vi "ICM Parsing Logic.vi"(8 "error in (no error)":errorcluster, 10 "Data String":string, 11 "Format String":string) -> (0 "error out":errorcluster, 3 "Data Values":dbl[](array[numeric]))   [LabVIEW 2018]
doc: "ICM Parsing Logic.vi\n\nThis VI includes the parsing functionality built into LabVIEW and custom parsing written for ICM. It is used by the ICM General Parser and the ICM Multi-Sentence Parser.\n\nInstrument Communication Module Version 1.0\nDecember, 2020 Original Code Consulting David Thomson\n www.originalcode.com"
uses:
  Parsing VIs/ICM whitespace.ctl
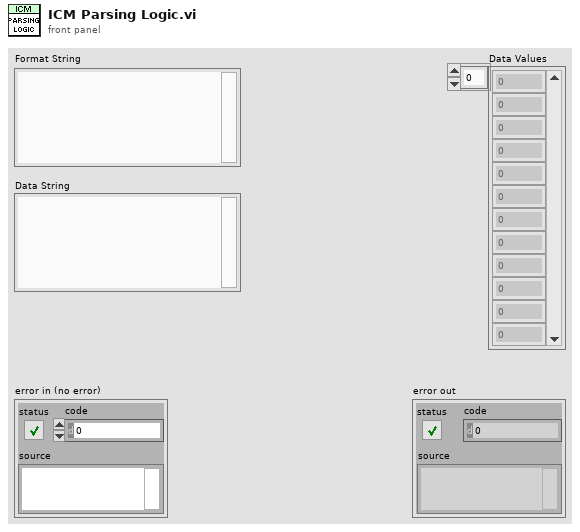
[diagram p1: front panel]
types:
  T1 = typedef "ICM whitespace.ctl" = u16
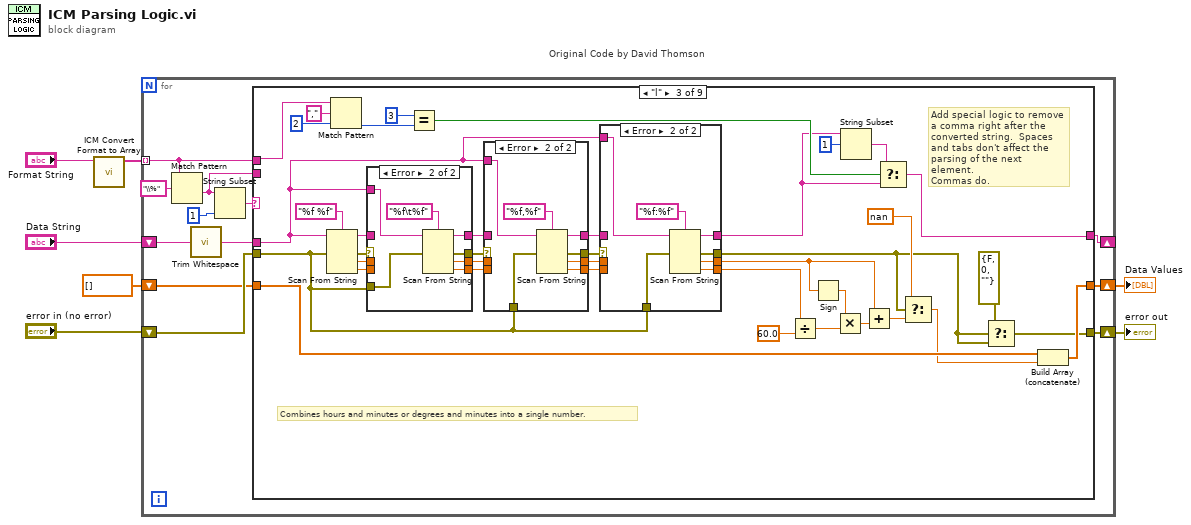
[diagram p0: block diagram]
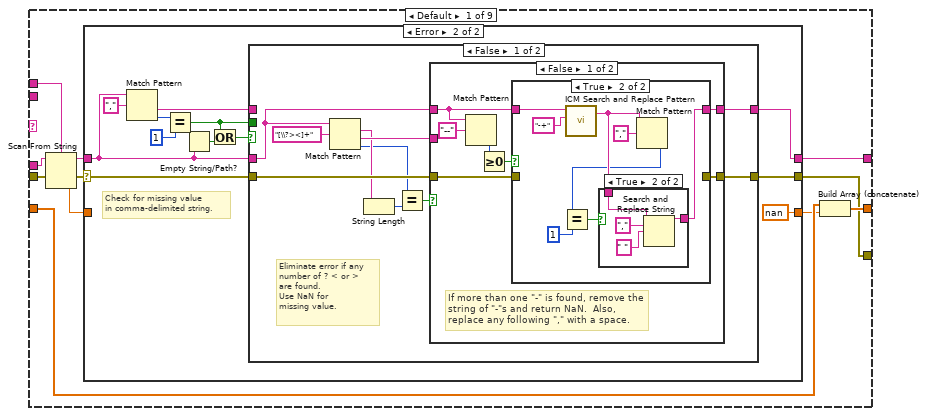
[diagram p2: hidden frame]
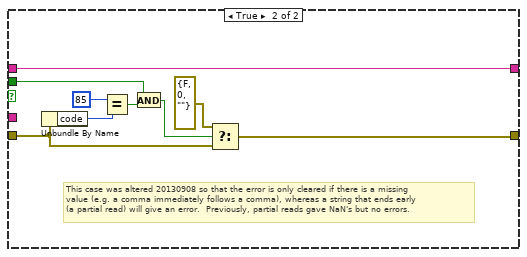
[diagram p7: hidden frame]
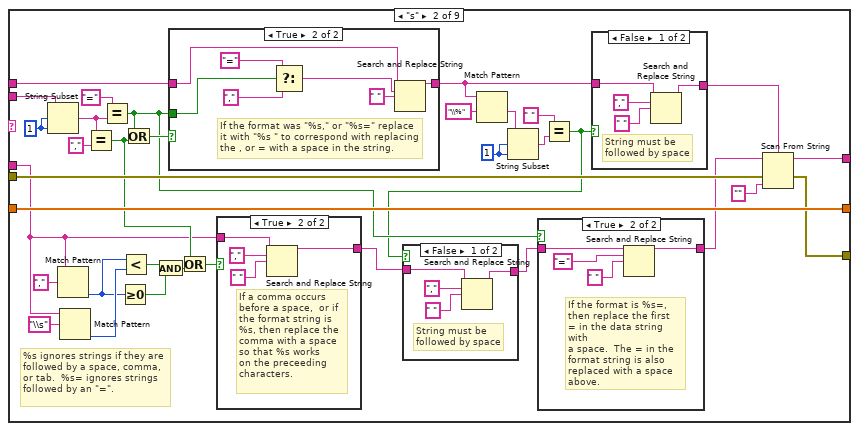
[diagram p8: hidden frame]
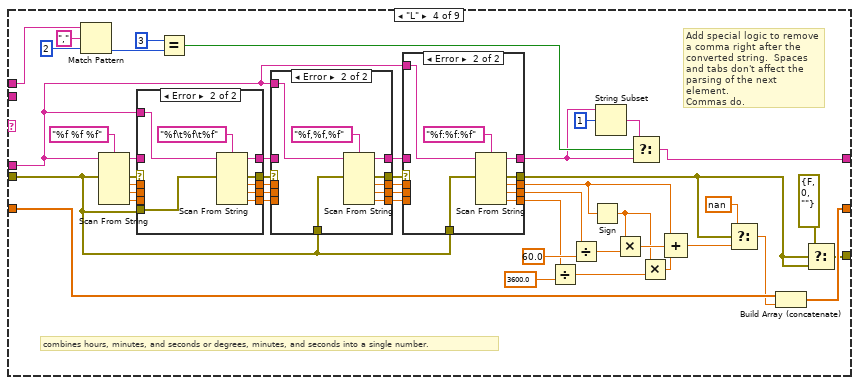
[diagram p17: hidden frame]
diagram:
  n1 = call "ICM Convert Format to Array.vi"("Format String"="Format String") -> ("Format Array"=w7:string[])  [unwired: 10 in]
  n2 = for "Original Code by David Thomson" {
    shift-right: [w13] -> _
    shift-left: "Data String" -> [w9]
    shift-right: [w14] -> w2
    shift-left: "error in (no error)" -> [w19]
    tunnel: w7 -> [w11] mode=indexing
    shift-right: [w16] -> w5
    shift-left: dbl[] [] -> [w17]
    n3 = Match Pattern(string=w11, regular expression="\\%") -> (after substring=w10:string)  [unwired: 4 out]
    n4 = call <vilib>:"Trim Whitespace.vi"("string"=w9) -> ("trimmed string"=w8:string)  [unwired: 1 in]
    n5 = String Subset(string=w10, length (rest)=1 ("length (rest)")) -> (substring=w15:string)  [unwired: 1 out]
    n6 = case shown="\"l\"" w15 {
      selector: w15 -> [_ _ _ _ _ w347 _ _ _]
      tunnel: w19 -> [w30 w118 w155 w230 w326 w355 w441 w459 w557]
      tunnel: w11 -> [w29 w108 w170 w240 _ _ _ _ _]
      tunnel: [w28 w119 w182 w262 w324 w339 w443 w460 w555] -> w16
      tunnel: w17 -> [w23 w119 w183 w263 w325 _ w443 w461 w572]
      tunnel: [w26 w117 w160 w234 w322 w348 w441 w458 w558] -> w14
      tunnel: [w21 w121 w165 w236 w323 w349 w442 w463 w551] -> w13
      tunnel: w10 -> [_ w110 _ _ w310 _ w437 w457 w565]
      tunnel: w8 -> [w20 w88 w150 w222 w307 w336 w429 w448 w550]
      frame Default {
        n7 = Scan From String(format string=w29, input string=w20, error in=w30) -> (remaining string=w25:string, error out=w27:errorcluster, output 1=w24:dbl)  [unwired: 1 in, 2 out]
        n8 = case shown="Error" w27 {
          selector: w27 -> [w33 w41]
          tunnel: [w33 w35] -> w26
          tunnel: [w32 w36] -> w21
          tunnel: w25 -> [w32 w37]
          tunnel: w24 -> [w31 _]
          tunnel: [w31 nan ("y")] -> w22
          frame No Error {
            # "this case uses LabVIEW's built in parsing codes"
          }
          frame Error {
            # "Check for missing value\nin comma-delimited string."
            n9 = Match Pattern(string=w37, regular expression=",") -> (after substring=w42:string, offset past match=w44:i32)  [unwired: 3 out]
            n10 = Equal?(x=w44, y=1) -> (x = y?=w34:bool)
            n11 = Empty String/Path?(string/path=w37) -> (empty?=w38:bool)
            n12 = Or(x=w34, y=w38) -> (x .or. y?=w39:bool)
            n13 = case shown="False" w39 {
              tunnel: [w51 w87] -> w36
              tunnel: w42 -> [_ w87]
              tunnel: w37 -> [w53 _]
              tunnel: [w50 w86] -> w35
              tunnel: w41 -> [w52 w85]
              tunnel: w34 -> [_ w80]
              frame False {
                # "Eliminate error if any\nnumber of ? < or >\nare found.\nUse NaN for\nmissing value."
                n14 = Match Pattern(string=w53, regular expression="[\\?><]+") -> (match substring=w48:string, after substring=w49:string, offset past match=w46:i32)  [unwired: 2 out]
                n15 = String Length(string=w48) -> (length=w47:i32)
                n16 = Equal?(x=w46, y=w47) -> (x = y?=w54:bool)
                n17 = case shown="False" w54 {
                  tunnel: [w57 w78] -> w51
                  tunnel: w53 -> [w56 _]
                  tunnel: [w58 _] -> w50
                  tunnel: w52 -> [w59 _]
                  tunnel: w49 -> [_ w78]
                  frame False {
                    # "If more than one \"-\" is found, remove the\nstring of \"-\"s and return NaN.  Also,\nreplace any following \",\" with a space."
                    n18 = Match Pattern(string=w56, regular expression="--") -> (offset past match=w61:i32)  [unwired: 4 out]
                    n19 = Greater Or Equal To 0?(x=w61) -> (x >= 0?=w60:bool)
                    n20 = case shown="True" w60 {
                      tunnel: [w64 _] -> w58
                      tunnel: w59 -> [w64 _]
                      tunnel: [w63 w70] -> w57
                      tunnel: w56 -> [w63 w72]
                      frame False {
                      }
                      frame True {
                        n21 = call "ICM Search and Replace Pattern.vi"("string"=w72, "regular expression (\"\")"="-+" ("regular expression (\"\")")) -> ("result string"=w68:string)  [unwired: 1 in, 3 out]
                        n22 = Match Pattern(string=w68, regular expression=",") -> (offset past match=w66:i32)  [unwired: 4 out]
                        n23 = Equal?(x=w66, y=1) -> (x = y?=w65:bool)
                        n24 = case shown="True" w65 {
                          tunnel: w68 -> [w73 w75]
                          tunnel: [w73 w74] -> w70
                          frame False {
                          }
                          frame True {
                            n25 = Search and Replace String(input string=w75, search string=",", replace string=" " ("replace string (\"\")")) -> (result string=w74:string)  [unwired: 1 in, 7 out]
                          }
                        }
                      }
                    }
                  }
                  frame True {
                  }
                }
              }
              frame True {
                # "This case was altered 20130908 so that the error is only cleared if there is a missing\nvalue (e.g. a comma immediately follows a comma), whereas a string that ends early\n(a partial read) will give an error.  Previously, partial reads gave NaN's but no errors."
                n26 = Unbundle By Name(w85) -> ("code"=w84:i32)
                n27 = Equal?(x=85, y=w84) -> (x = y?=w81:bool)
                n28 = And(x=w80, y=w81) -> (x .and. y?=w79:bool)
                n29 = Select(t=errorcluster {"status"=FALSE, "code"=0, "source"=""}, s=w79, f=w85) -> (s? t:f=w86:errorcluster)
              }
            }
          }
        }
        n30 = Build Array (concatenate)(w23, w22) -> (w28:dbl[])
      }
      frame "s" {
        w94 = 1 ("length (rest)")
        w107 = 1 ("length (rest)")
        # "%s ignores strings if they are\nfollowed by a space, comma,\nor tab.  %s= ignores strings followed by an \"=\"."
        n31 = String Subset(string=w110, offset (0)=w107, length (rest)=w107) -> (substring=w105:string)
        n32 = Match Pattern(string=w88, regular expression=",") -> (offset past match=w112:i32)  [unwired: 4 out]
        n33 = Match Pattern(string=w88, regular expression="\\s") -> (offset past match=w114:i32)  [unwired: 4 out]
        n34 = Equal?(x=w105, y=",") -> (x = y?=w100:bool)
        n35 = Equal?(x="=" ("y"), y=w105) -> (x = y?=w102:bool)
        n36 = Greater Or Equal To 0?(x=w112) -> (x >= 0?=w111:bool)
        n37 = Less?(x=w112, y=w114) -> (x < y?=w113:bool)
        n38 = Or(x=w102, y=w100) -> (x .or. y?=w106:bool)
        n39 = And(x=w113, y=w111) -> (x .and. y?=w101:bool)
        n40 = case shown="True" w106 {
          tunnel: [w137 w142] -> w93
          tunnel: w108 -> [w137 w143]
          tunnel: w102 -> [_ w138]
          frame False {
          }
          frame True {
            # "If the format was \"%s,\" or \"%s=\" replace\nit with \"%s \" to correspond with replacing\nthe , or = with a space in the string."
            n41 = Select(t="=" ("y"), s=w138, f="," ("search string")) -> (s? t:f=w139:string)
            n42 = Search and Replace String(input string=w143, search string=w139, replace string=" " ("replace string (\"\")")) -> (result string=w142:string)  [unwired: 1 in, 7 out]
          }
        }
        n43 = Or(x=w100, y=w101) -> (x .or. y?=w99:bool)
        n44 = case shown="True" w99 {
          tunnel: [w145 w147] -> w91
          tunnel: w88 -> [w145 w146]
          frame False {
          }
          frame True {
            # "If a comma occurs\nbefore a space,  or if\nthe format string is %s, then replace the comma with a space so that %s works\non the preceeding characters."
            n45 = Search and Replace String(input string=w146, search string=",", replace string=" " ("replace string (\"\")")) -> (result string=w147:string)  [unwired: 1 in, 7 out]
          }
        }
        n46 = Match Pattern(string=w93, regular expression="\\%") -> (after substring=w95:string)  [unwired: 4 out]
        n47 = String Subset(string=w95, offset (0)=w94, length (rest)=w94) -> (substring=w96:string)
        n48 = Equal?(x=" " ("y"), y=w96) -> (x = y?=w89:bool)
        n49 = case shown="False" w89 {
          tunnel: w91 -> [w123 w126]
          tunnel: [w122 w126] -> w90
          frame False {
            # "String must be \nfollowed by space"
            n50 = Search and Replace String(input string=w123, search string=",", replace string=" " ("replace string (\"\")")) -> (result string=w122:string)  [unwired: 1 in, 7 out]
          }
          frame True {
          }
        }
        n51 = case shown="True" w102 {
          tunnel: w90 -> [w132 w134]
          tunnel: [w132 w133] -> w103
          frame False {
          }
          frame True {
            # "If the format is %s=,\nthen replace the first\n= in the data string with\na space.  The = in the\nformat string is also\nreplaced with a space\nabove."
            n52 = Search and Replace String(input string=w134, search string="=", replace string=" " ("replace string (\"\")")) -> (result string=w133:string)  [unwired: 1 in, 7 out]
          }
        }
        n53 = case shown="False" w89 {
          tunnel: w93 -> [w128 w131]
          tunnel: [w127 w131] -> w92
          frame False {
            # "String must be \nfollowed by space"
            n54 = Search and Replace String(input string=w128, search string=",", replace string=" " ("replace string (\"\")")) -> (result string=w127:string)  [unwired: 1 in, 7 out]
          }
          frame True {
          }
        }
        n55 = Scan From String(format string=w92, input string=w103, error in=w118, default 1="") -> (remaining string=w121:string, error out=w117:errorcluster)  [unwired: 1 in, 2 out]
      }
      frame "l" {
        # "Combines hours and minutes or degrees and minutes into a single number."
        # "Add special logic to remove\na comma right after the\nconverted string.  Spaces\nand tabs don't affect the\nparsing of the next element.\nCommas do."
        n56 = Scan From String(format string="%f %f", input string=w150, error in=w155) -> (remaining string=w178:string, error out=w181:errorcluster, output 1=w180:dbl, output 2=w179:dbl)  [unwired: 1 in, 3 out]
        n57 = Match Pattern(string=w170, regular expression=",", offset (0)=2) -> (offset past match=w164:i32)  [unwired: 3 out]
        n58 = case shown="Error" w181 {
          selector: w181 -> [w214 _]
          tunnel: [w214 w215] -> w177
          tunnel: [w213 w220] -> w176
          tunnel: w180 -> [w213 _]
          tunnel: [w212 w219] -> w175
          tunnel: w179 -> [w212 _]
          tunnel: w178 -> [w211 _]
          tunnel: [w211 w218] -> w174
          tunnel: w150 -> [_ w217]
          tunnel: w155 -> [_ w216]
          frame No Error {
          }
          frame Error {
            n59 = Scan From String(format string="%f\t%f", input string=w217, error in=w216) -> (remaining string=w218:string, error out=w215:errorcluster, output 1=w220:dbl, output 2=w219:dbl)  [unwired: 1 in, 3 out]
          }
        }
        n60 = Equal?(x=3, y=w164) -> (x = y?=w163:bool)
        n61 = case shown="Error" w177 {
          selector: w177 -> [w203 _]
          tunnel: [w203 w207] -> w158
          tunnel: [w202 w209] -> w157
          tunnel: w176 -> [w202 _]
          tunnel: [w201 w208] -> w156
          tunnel: w175 -> [w201 _]
          tunnel: w174 -> [w200 _]
          tunnel: [w200 w206] -> w159
          tunnel: w150 -> [_ w205]
          tunnel: w155 -> [_ w204]
          frame No Error {
          }
          frame Error {
            n62 = Scan From String(format string="%f,%f", input string=w205, error in=w204) -> (remaining string=w206:string, error out=w207:errorcluster, output 1=w209:dbl, output 2=w208:dbl)  [unwired: 1 in, 3 out]
          }
        }
        n63 = case shown="Error" w158 {
          selector: w158 -> [w192 _]
          tunnel: [w192 w196] -> w153
          tunnel: [w191 w198] -> w152
          tunnel: w157 -> [w191 _]
          tunnel: [w190 w197] -> w151
          tunnel: w156 -> [w190 _]
          tunnel: w159 -> [w189 _]
          tunnel: [w189 w195] -> w154
          tunnel: w150 -> [_ w194]
          tunnel: w155 -> [_ w193]
          frame No Error {
          }
          frame Error {
            n64 = Scan From String(format string="%f:%f", input string=w194, error in=w193) -> (remaining string=w195:string, error out=w196:errorcluster, output 1=w198:dbl, output 2=w197:dbl)  [unwired: 1 in, 3 out]
          }
        }
        n65 = Divide(x=w151, y=60.0) -> (x/y=w186:dbl)
        n66 = Sign(1:w152) -> (0:w185:dbl)
        n67 = Multiply(x=w185, y=w186) -> (x*y=w184:dbl)
        n68 = String Subset(string=w154, offset (0)=1) -> (substring=w166:string)  [unwired: 1 out]
        n69 = Add(x=w152, y=w184) -> (x+y=w173:dbl)
        n70 = Select(t=w166, s=w163, f=w154) -> (s? t:f=w165:string)
        n71 = Select(t=nan ("y"), s=w153, f=w173) -> (s? t:f=w172:dbl)
        n72 = Select(t=errorcluster {"status"=FALSE, "code"=0, "source"=""}, s=w153, f=w153) -> (s? t:f=w160:errorcluster)
        n73 = Build Array (concatenate)(w183, w172) -> (w182:dbl[])
      }
      frame "L" {
        # "combines hours, minutes, and seconds or degrees, minutes, and seconds into a single number."
        # "Add special logic to remove\na comma right after the\nconverted string.  Spaces\nand tabs don't affect the\nparsing of the next element.\nCommas do."
        n74 = Match Pattern(string=w240, regular expression=",", offset (0)=2) -> (offset past match=w242:i32)  [unwired: 3 out]
        n75 = Scan From String(format string="%f %f %f", input string=w222, error in=w230) -> (remaining string=w258:string, error out=w261:errorcluster, output 1=w260:dbl, output 2=w259:dbl, output 3=w250:dbl)  [unwired: 1 in, 4 out]
        n76 = case shown="Error" w261 {
          selector: w261 -> [w298 _]
          tunnel: [w298 w300] -> w257
          tunnel: [w297 w305] -> w256
          tunnel: w260 -> [w297 _]
          tunnel: [w296 w304] -> w255
          tunnel: w259 -> [w296 _]
          tunnel: w258 -> [w295 _]
          tunnel: [w295 w303] -> w254
          tunnel: w222 -> [_ w302]
          tunnel: w230 -> [_ w301]
          tunnel: w250 -> [w294 _]
          tunnel: [w294 w299] -> w249
          frame No Error {
          }
          frame Error {
            n77 = Scan From String(format string="%f\t%f\t%f", input string=w302, error in=w301) -> (remaining string=w303:string, error out=w300:errorcluster, output 1=w305:dbl, output 2=w304:dbl, output 3=w299:dbl)  [unwired: 1 in, 4 out]
          }
        }
        n78 = Equal?(x=3, y=w242) -> (x = y?=w237:bool)
        n79 = case shown="Error" w257 {
          selector: w257 -> [w285 _]
          tunnel: [w285 w290] -> w223
          tunnel: [w284 w292] -> w228
          tunnel: w256 -> [w284 _]
          tunnel: [w283 w291] -> w226
          tunnel: w255 -> [w283 _]
          tunnel: w254 -> [w282 _]
          tunnel: [w282 w289] -> w233
          tunnel: w222 -> [_ w288]
          tunnel: w230 -> [_ w287]
          tunnel: [w281 w286] -> w227
          tunnel: w249 -> [w281 _]
          frame No Error {
          }
          frame Error {
            n80 = Scan From String(format string="%f,%f,%f", input string=w288, error in=w287) -> (remaining string=w289:string, error out=w290:errorcluster, output 1=w292:dbl, output 2=w291:dbl, output 3=w286:dbl)  [unwired: 1 in, 4 out]
          }
        }
        n81 = case shown="Error" w223 {
          selector: w223 -> [w272 _]
          tunnel: [w272 w277] -> w225
          tunnel: [w271 w279] -> w229
          tunnel: w228 -> [w271 _]
          tunnel: [w270 w278] -> w231
          tunnel: w226 -> [w270 _]
          tunnel: w233 -> [w269 _]
          tunnel: [w269 w276] -> w224
          tunnel: w222 -> [_ w275]
          tunnel: w230 -> [_ w274]
          tunnel: [w268 w273] -> w232
          tunnel: w227 -> [w268 _]
          frame No Error {
          }
          frame Error {
            n82 = Scan From String(format string="%f:%f:%f", input string=w275, error in=w274) -> (remaining string=w276:string, error out=w277:errorcluster, output 1=w279:dbl, output 2=w278:dbl, output 3=w273:dbl)  [unwired: 1 in, 4 out]
          }
        }
        n83 = Divide(x=w232, y=3600.0) -> (x/y=w248:dbl)
        n84 = Divide(x=w231, y=60.0) -> (x/y=w265:dbl)
        n85 = Sign(1:w229) -> (0:w246:dbl)
        n86 = String Subset(string=w224, offset (0)=1) -> (substring=w238:string)  [unwired: 1 out]
        n87 = Multiply(x=w246, y=w265) -> (x*y=w264:dbl)
        n88 = Select(t=w238, s=w237, f=w224) -> (s? t:f=w236:string)
        n89 = Multiply(x=w246, y=w248) -> (x*y=w245:dbl)
        n90 = Compound Arithmetic op=ADD(w229, w264, w245) -> (w253:dbl)
        n91 = Select(t=nan ("y"), s=w225, f=w253) -> (s? t:f=w252:dbl)
        n92 = Build Array (concatenate)(w263, w252) -> (w262:dbl[])
        n93 = Select(t=errorcluster {"status"=FALSE, "code"=0, "source"=""}, s=w225, f=w225) -> (s? t:f=w234:errorcluster)
      }
      frame "q" {
        w312 = 1 ("length (rest)")
        # "Convert month string to number (Jan = 1)"
        n94 = String Subset(string=w310, offset (0)=w312, length (rest)=w312) -> (substring=w311:string)
        n95 = Equal?(x=w311, y=",") -> (x = y?=w309:bool)
        n96 = case shown="True" w309 {
          tunnel: w307 -> [w331 w333]
          tunnel: [w331 w332] -> w308
          frame False {
          }
          frame True {
            # "If the format is \"%q,\" then\nreplace the first , in the data\nstring with a space."
            n97 = Search and Replace String(input string=w333, search string=",", replace string=" " ("replace string (\"\")")) -> (result string=w332:string)  [unwired: 1 in, 7 out]
          }
        }
        n98 = Scan From String(format string="%s", input string=w308, error in=w326) -> (remaining string=w323:string, error out=w322:errorcluster, output 1=w321:string)  [unwired: 1 in, 2 out]
        n99 = String Subset(string=w321, length (rest)=3 ("length (rest)")) -> (substring=w319:string)  [unwired: 1 out]
        n100 = To Upper Case(1:w319) -> (0:w328:string)
        n101 = Search 1D Array(1D array=string[] ["JAN", "FEB", "MAR", "APR", "MAY", "JUN", "JUL", "AUG", "SEP", "OCT", "NOV", "DEC"], element=w328) -> (index of element=w330:i32)  [unwired: 1 out]
        n102 = Increment(x=w330) -> (x+1=w318:i32)
        n103 = Equal To 0?(x=w318) -> (x = 0?=w317:bool)
        n104 = To Double Precision Float(number=w318) -> (double precision float=w316:dbl)
        n105 = Select(t=nan ("y"), s=w317, f=w316) -> (s? t:f=w315:dbl)
        n106 = Build Array (concatenate)(w325, w315) -> (w324:dbl[])
      }
      frame "I", "i" {
        w337 = T1 1 items=["both", "start of string", "end of string"] ("location (both)")
        # "decodes ISO 8601 time strings\n\"I\" includes a time stamp before\nthe other channels"
        n107 = call "ICM Trim Whitespace.vi"("string"=w336, "location (both)"=w337) -> ("trimmed string"=w338:string)
        n108 = Match Pattern(string=w338, regular expression="[T\\s]") -> (before substring=w356:string, after substring=w351:string)  [unwired: 3 out]
        n109 = Match Pattern(string=w351, regular expression="[\\s\\t,]") -> (before substring=w350:string, after substring=w349:string)  [unwired: 3 out]
        n110 = Match Pattern(string=w356, regular expression="-") -> (offset past match=w357:i32)  [unwired: 4 out]
        n111 = case "Decode Date" shown="5" w357 {
          tunnel: w356 -> [w415 w428]
          tunnel: [w412 w425] -> w341
          tunnel: [w407 w424] -> w340
          tunnel: [w413 w426] -> w342
          tunnel: w355 -> [w406 w422]
          tunnel: [w403 w421] -> w343
          frame 0, Default {
            w409 = 0.0 ("default value 1")
            w408 = "%d" ("format string")
            n112 = String Subset(string=w415, length (rest)=4 ("length (rest)")) -> (substring=w414:string)  [unwired: 1 out]
            n113 = String Subset(string=w415, offset (0)=4, length (rest)=2 ("length (rest)")) -> (substring=w411:string)
            n114 = String Subset(string=w415, offset (0)=6, length (rest)=2 ("length (rest)")) -> (substring=w410:string)
            n115 = Scan From String(format string=w408, input string=w410, error in=w406, default 1=w409) -> (error out=w405:errorcluster, output 1=w407:dbl)  [unwired: 1 in, 2 out]
            n116 = Scan From String(format string=w408, input string=w411, error in=w405, default 1=w409) -> (error out=w404:errorcluster, output 1=w412:dbl)  [unwired: 1 in, 2 out]
            n117 = Scan From String(format string=w408, input string=w414, error in=w404, default 1=w409) -> (error out=w403:errorcluster, output 1=w413:dbl)  [unwired: 1 in, 2 out]
          }
          frame 5 {
            w423 = 0.0 ("default value 1")
            n118 = Scan From String(format string="%d-%d-%d", input string=w428, error in=w422, default 1=w423, default 2=w423, default 3=w423) -> (error out=w421:errorcluster, output 1=w426:dbl, output 2=w425:dbl, output 3=w424:dbl)  [unwired: 1 in, 2 out]
          }
        }
        n119 = Match Pattern(string=w350, regular expression=":") -> (offset past match=w353:i32)  [unwired: 4 out]
        n120 = case "Decode Time" shown="3" w353 {
          tunnel: w350 -> [w389 w402]
          tunnel: [w387 w399] -> w345
          tunnel: [w382 w398] -> w344
          tunnel: [w376 w400] -> w346
          tunnel: w343 -> [w381 w396]
          tunnel: [w378 w395] -> w348
          frame 0, Default {
            w384 = 0.0 ("default value 1")
            w383 = "%d" ("format string")
            n121 = String Subset(string=w389, length (rest)=2 ("length (rest)")) -> (substring=w388:string)  [unwired: 1 out]
            n122 = String Subset(string=w389, offset (0)=2, length (rest)=2 ("length (rest)")) -> (substring=w386:string)
            n123 = String Subset(string=w389, offset (0)=4, length (rest)=2 ("length (rest)")) -> (substring=w385:string)
            n124 = Scan From String(format string="%f", input string=w385, error in=w381, default 1=w384) -> (error out=w380:errorcluster, output 1=w382:dbl)  [unwired: 1 in, 2 out]
            n125 = Scan From String(format string=w383, input string=w386, error in=w380, default 1=w384) -> (error out=w379:errorcluster, output 1=w387:dbl)  [unwired: 1 in, 2 out]
            n126 = Scan From String(format string=w383, input string=w388, error in=w379, default 1=w384) -> (error out=w378:errorcluster, output 1=w376:dbl)  [unwired: 1 in, 2 out]
          }
          frame 3 {
            w397 = 0.0 ("default value 1")
            n127 = Scan From String(format string="%d:%d:%f", input string=w402, error in=w396, default 1=w397, default 2=w397, default 3=w397) -> (error out=w395:errorcluster, output 1=w400:dbl, output 2=w399:dbl, output 3=w398:dbl)  [unwired: 1 in, 2 out]
          }
        }
        n128 = case shown="\"I\"" w347 {
          tunnel: w346 -> [w363 w375]
          tunnel: w345 -> [w362 w370]
          tunnel: w344 -> [w361 w371]
          tunnel: w342 -> [w366 w367]
          tunnel: w341 -> [w365 w368]
          tunnel: w340 -> [w364 w369]
          tunnel: [w360 w374] -> w339
          frame "i", Default {
            n129 = Build Array(w366, w365, w364, w363, w362, w361) -> (w360:dbl[])
          }
          frame "I" {
            n130 = call "ICM Calculate Time Stamps.vi"("Second"=w371, "Year"=w367, "Minute"=w370, "Hour"=w370, "Day"=w369, "Month"=w368) -> ("Seconds Since Midnight"=w373:dbl, "TimeStamp"=w372:dbl)  [unwired: 4 in]
            n131 = Build Array(w372, w373, w367, w368, w369, w375, w370, w371) -> (w374:dbl[])
          }
        }
      }
      frame "z" {
        w434 = "," ("regular expression")
        # "special case for %z with no \"n\" following it - skip one character"
        # "%zn ignores n characters"
        n132 = Match Pattern(string=w437, regular expression=w434) -> (before substring=w436:string, match substring=w435:string)  [unwired: 3 out]
        n133 = Equal?(x=w435, y=w434) -> (x = y?=w432:bool)
        n134 = String Length(string=w436) -> (length=w439:i32)
        n135 = Greater?(x=w439, y=1) -> (0:w440:bool)
        n136 = case shown="True" w440 {
          tunnel: w436 -> [_ w447]
          tunnel: [1 w445] -> w431
          frame False {
          }
          frame True {
            n137 = Scan From String(format string="z%d", input string=w447) -> (output 1=w445:i32)  [unwired: 2 in, 4 out]
          }
        }
        n138 = Increment(x=w431) -> (x+1=w430:i32)
        n139 = Select(t=w430, s=w432, f=w431) -> (s? t:f=w433:i32)
        n140 = String Subset(string=w429, offset (0)=w433) -> (substring=w442:string)  [unwired: 1 out]
      }
      frame "a" {
        # "parse binary data"
        n141 = String Subset(string=w457, offset (0)=1) -> (substring=w456:string)  [unwired: 1 out]
        n142 = Match Pattern(string=w456, regular expression="-") -> (after substring=w464:string, offset past match=w465:i32)  [unwired: 3 out]
        n143 = Greater Or Equal To 0?(x=w465) -> (x >= 0?=w462:bool)
        n144 = Select(t=w464, s=w462, f=w456) -> (s? t:f=w450:string)
        n145 = Match Pattern(string=w450, regular expression="\\^") -> (after substring=w453:string, offset past match=w451:i32)  [unwired: 3 out]
        n146 = Greater Or Equal To 0?(x=w451) -> (x >= 0?=w449:bool)
        n147 = Select(t=w453, s=w449, f=w450) -> (s? t:f=w452:string)
        n148 = case shown="\"U8\"" w452 {
          tunnel: w448 -> [w471 w477 w486 w494 w502 w508 w517 w525 w533 w541 w549]
          tunnel: [w471 w476 w485 w493 w501 w507 w516 w524 w532 w540 w548] -> w463
          tunnel: w462 -> [_ _ w480 w492 w500 _ w511 w523 w531 w539 w547]
          tunnel: w461 -> [w470 w475 w484 w491 w499 w506 w515 w522 w530 w538 w546]
          tunnel: [w470 w473 w482 w489 w497 w504 w513 w520 w528 w536 w544] -> w460
          tunnel: [w469 w472 w481 w488 w496 w503 w512 w519 w527 w535 w543] -> w458
          tunnel: w459 -> [w468 w472 w481 w488 w496 w503 w512 w519 w527 w535 w543]
          tunnel: w449 -> [_ _ w479 w487 w495 _ w510 w518 w526 w534 w542]
          frame "", Default {
            n149 = call "Error Cluster Generator.vi"("error in"=w468, "code"=82) -> ("error out"=w469:errorcluster)  [unwired: 4 in, 1 out]
          }
          frame "U8" {
            n150 = call "ICM aU8.vi"("String In"=w477) -> ("Value"=w474:dbl, "String Out"=w476:string)  [unwired: 1 in, 8 out]
            n151 = Build Array (concatenate)(w475, w474) -> (w473:dbl[])
          }
          frame "U16" {
            n152 = Or(x=w479, y=w480) -> (x .or. y?=w478:bool)
            n153 = call "ICM aU16.vi"("Reverse Bytes"=w478, "String In"=w486) -> ("Value"=w483:dbl, "String Out"=w485:string)  [unwired: 8 out]
            n154 = Build Array (concatenate)(w484, w483) -> (w482:dbl[])
          }
          frame "U32" {
            n155 = call "ICM aU32.vi"("Reverse Bytes"=w492, "Swap Bytes"=w487, "String In"=w494) -> ("Value"=w490:dbl, "String Out"=w493:string)  [unwired: 1 in, 6 out]
            n156 = Build Array (concatenate)(w491, w490) -> (w489:dbl[])
          }
          frame "U64" {
            n157 = call "ICM aU64.vi"("Reverse Bytes"=w500, "Swap Bytes"=w495, "String In"=w502) -> ("Value"=w498:dbl, "String Out"=w501:string)  [unwired: 7 out]
            n158 = Build Array (concatenate)(w499, w498) -> (w497:dbl[])
          }
          frame "I8" {
            n159 = call "ICM aI8.vi"("String In"=w508) -> ("Value"=w505:dbl, "String Out"=w507:string)  [unwired: 1 in, 8 out]
            n160 = Build Array (concatenate)(w506, w505) -> (w504:dbl[])
          }
          frame "I16" {
            n161 = Or(x=w510, y=w511) -> (x .or. y?=w509:bool)
            n162 = call "ICM aI16.vi"("Swap Bytes"=w509, "String In"=w517) -> ("Value"=w514:dbl, "String Out"=w516:string)  [unwired: 8 out]
            n163 = Build Array (concatenate)(w515, w514) -> (w513:dbl[])
          }
          frame "I32" {
            n164 = call "ICM aI32.vi"("Reverse Bytes"=w523, "Swap Bytes"=w518, "String In"=w525) -> ("Value"=w521:dbl, "String Out"=w524:string)  [unwired: 7 out]
            n165 = Build Array (concatenate)(w522, w521) -> (w520:dbl[])
          }
          frame "I64" {
            n166 = call "ICM aI64.vi"("Reverse Bytes"=w531, "Swap Bytes"=w526, "String In"=w533) -> ("Value"=w529:dbl, "String Out"=w532:string)  [unwired: 7 out]
            n167 = Build Array (concatenate)(w530, w529) -> (w528:dbl[])
          }
          frame "SGL" {
            n168 = call "ICM aSGL.vi"("Reverse Bytes"=w539, "Swap Bytes"=w534, "String In"=w541) -> ("Value"=w537:dbl, "String Out"=w540:string)  [unwired: 7 out]
            n169 = Build Array (concatenate)(w538, w537) -> (w536:dbl[])
          }
          frame "DBL" {
            n170 = call "ICM aDBL.vi"("Reverse Bytes"=w547, "Swap Bytes"=w542, "String In"=w549) -> ("Value"=w545:dbl, "String Out"=w548:string)  [unwired: 7 out]
            n171 = Build Array (concatenate)(w546, w545) -> (w544:dbl[])
          }
        }
      }
      frame "c" {
        # "scale the previous channel by a polynomial"
        n172 = Delete From Array(array=w572) -> (deleted portion=w553:dbl, array with subset deleted=w556:dbl[])  [unwired: 2 in]
        n173 = Match Pattern(string=w565, regular expression="\\[", offset (0)=1) -> (after substring=w571:string, offset past match=w563:i32)  [unwired: 2 out]
        n174 = Match Pattern(string=w571, regular expression="\\]") -> (before substring=w569:string, offset past match=w561:i32)  [unwired: 3 out]
        n175 = Spreadsheet String To Array(delimiter (Tab)=",", format string="%f", spreadsheet string=w569, array type (2D Dbl)=dbl[] []) -> (array=w554:dbl[])
        n176 = Less Than 0?(x=w563) -> (x < 0?=w562:bool)
        n177 = Less Than 0?(x=w561) -> (x < 0?=w560:bool)
        n178 = Or(x=w562, y=w560) -> (x .or. y?=w559:bool)
        n179 = case shown="False" w559 {
          tunnel: [w580 w591] -> w558
          tunnel: w557 -> [w580 w590]
          tunnel: [w579 w589] -> w555
          tunnel: w556 -> [w578 w589]
          tunnel: w550 -> [w577 w588]
          tunnel: [w577 w588] -> w551
          tunnel: w554 -> [w576 _]
          tunnel: w553 -> [w575 _]
          frame False {
            n180 = for {
              tunnel: w576 -> [w587] mode=indexing
              tunnel: w575 -> [w583]
              shift-right: [w586] -> w573
              shift-left: 0.0 ("Numeric") -> [w584]
              i -> [w582]
              n181 = Power Of X(1:w583, 2:w582) -> (0:w581:dbl)
              n182 = Multiply(x=w587, y=w581) -> (x*y=w585:dbl)
              n183 = Add(x=w585, y=w584) -> (x+y=w586:dbl)
            }
            n184 = Build Array (concatenate)(w578, w573) -> (w579:dbl[])
          }
          frame True {
            n185 = call "Error Cluster Generator.vi"("error in"=w590, "code"=82) -> ("error out"=w591:errorcluster)  [unwired: 2 in, 3 out]
          }
        }
      }
    }
  }
  "Data Values" <- w5
  "error out" <- w2
